vi "files_select.vi"(1 "right":path, 2 "left":path) -> (0 "Array":string[][](array[string]))   [LabVIEW 2010]
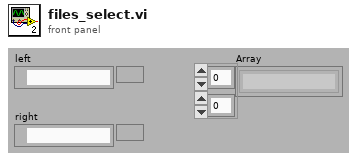
[diagram p1: front panel]
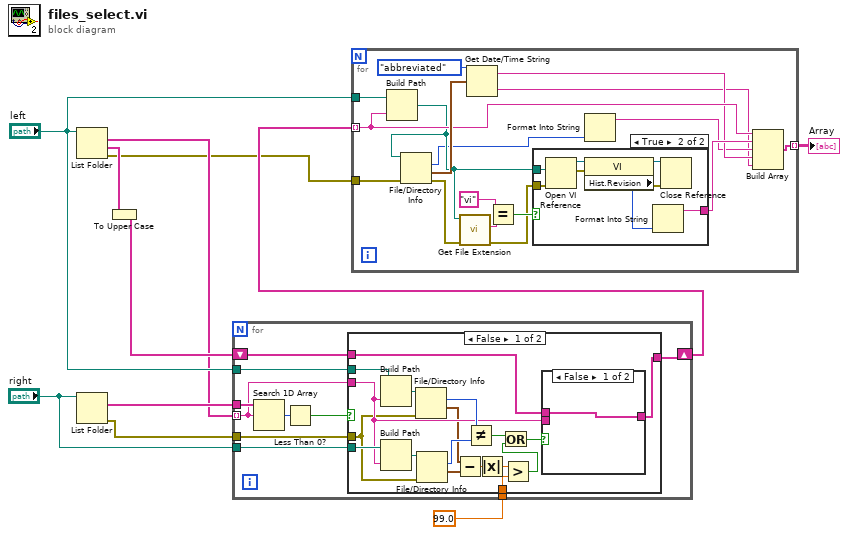
[diagram p0: block diagram]
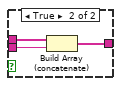
[diagram p2: hidden frame]
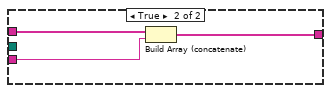
[diagram p3: hidden frame]
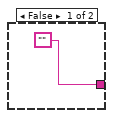
[diagram p4: hidden frame]
diagram:
  n1 = List Folder(path="left") -> (filenames=w5:string[], folder names=w6:string[], error out=w3:errorcluster)  [unwired: 3 in, 1 out]
  n2 = List Folder(path="right") -> (filenames=w10:string[], error out=w2:errorcluster)  [unwired: 3 in, 2 out]
  n3 = To Upper Case(1:w6) -> (0:w8:string[])
  n4 = for {
    tunnel: w5 -> [w18] mode=indexing
    tunnel: w10 -> [w21]
    shift-right: [w17] -> w7
    shift-left: w8 -> [w16]
    tunnel: "left" -> [w15]
    tunnel: "right" -> [w14]
    tunnel: w2 -> [w13]
    tunnel: 99.0 -> [w12]
    n5 = Search 1D Array(1D array=w21, element=w18) -> (index of element=w20:i32)  [unwired: 1 in]
    n6 = Less Than 0?(x=w20) -> (x < 0?=w19:bool)
    n7 = case shown="False" w19 {
      tunnel: w18 -> [w30 w46]
      tunnel: [w29 w45] -> w17
      tunnel: w16 -> [w31 w44]
      tunnel: w15 -> [w39 _]
      tunnel: w14 -> [w38 _]
      tunnel: w13 -> [w28 _]
      tunnel: w12 -> [w22 _]
      frame False {
        n8 = Build Path(base path=w39, name or relative path=w30) -> (appended path=w37:path)
        n9 = Build Path(base path=w38, name or relative path=w30) -> (appended path=w36:path)
        n10 = File/Directory Info(path=w37, error in=w28) -> (size=w35:i64, last mod=w27:timestamp)  [unwired: 5 out]
        n11 = File/Directory Info(path=w36, error in=w28) -> (size=w34:i64, last mod=w26:timestamp)  [unwired: 5 out]
        n12 = Subtract(x=w27, y=w26) -> (x-y=w25:dbl)
        n13 = Not Equal?(x=w35, y=w34) -> (x != y?=w33:bool)
        n14 = Absolute Value(x=w25) -> (abs(x)=w24:dbl)
        n15 = Greater?(x=w24, y=w22) -> (0:w23:bool)
        n16 = Or(x=w33, y=w23) -> (x .or. y?=w32:bool)
        n17 = case shown="False" w32 {
          tunnel: w31 -> [w40 w43]
          tunnel: w30 -> [_ w42]
          tunnel: [w40 w41] -> w29
          frame False {
          }
          frame True {
            n18 = Build Array (concatenate)(w43, w42) -> (w41:string[])
          }
        }
      }
      frame True {
        n19 = Build Array (concatenate)(w44, w46) -> (w45:string[])
      }
    }
  }
  n20 = for {
    tunnel: "left" -> [w63]
    tunnel: w3 -> [w60]
    tunnel: w7 -> [w59] mode=indexing
    tunnel: [w56] -> w4 mode=indexing
    n21 = Build Path(base path=w63, name or relative path=w59) -> (appended path=w55:path)
    n22 = File/Directory Info(path=w55, error in=w60) -> (size=w49:i64, last mod=w62:timestamp, error out=w54:errorcluster)  [unwired: 4 out]
    n23 = call <vilib>:"Get File Extension.vi"("error in (no error)"=w54, "file"=w55) -> ("error out"=w50:errorcluster, "lowercase file extension"=w53:string)  [unwired: 6 in, 2 out]
    n24 = Get Date/Time String(date format (0)=enum16{"short", "long", "abbreviated"}."abbreviated", seconds (now)=w62) -> (date string=w57:string, time string=w47:string)  [unwired: 1 in]
    n25 = Equal?(x="vi" ("pattern"), y=w53) -> (x = y?=w51:bool)
    n26 = case shown="True" w51 {
      tunnel: ["" w67] -> w58
      tunnel: w55 -> [_ w66]
      tunnel: w50 -> [_ w65]
      frame False {
      }
      frame True {
        n27 = Open VI Reference(vi path=w66, error in (no error)=w65) -> (vi reference=w71:refnum<vi>, error out=w72:errorcluster)  [unwired: 4 in]
        n28 = property class="VI"(reference=w71, error in=w72) -> (reference out=w70:refnum<vi>, error out=w69:errorcluster, "Hist.Revision"=w68:u32)
        n29 = Format Into String(w68) -> (resulting string=w67:string)  [unwired: 3 in, 1 out]
        n30 = Close Reference(reference=w70, error in (no error)=w69) -> ()  [unwired: 1 out]
      }
    }
    n31 = Format Into String(w49) -> (resulting string=w48:string)  [unwired: 3 in, 1 out]
    n32 = Build Array(w59, w58, w48, w57, w47) -> (w56:string[])
  }
  "Array" <- w4
